vi "CustomEventHandler.vi"(11 "MicronGRPC.lvclass":refnum<class "MicronGRPC.lvclass">) -> ()   [LabVIEW 2019, in "MicronGRPCGeneratedServer.lvlib"]
uses:
  MicronGRPCGeneratedServer.lvlib
  RPC Service/MicronGRPC/MicronGRPC.lvclass
  Message/GRPCMessage.lvclass
  D:/GitHub/KarthikAbiram/Micron/LabVIEW/Source/vi.lib/Micron/Base/Server/Message/MessageBase.lvclass
  <vilib>/SLL Toolkit/SLL String/SLL String.lvlib
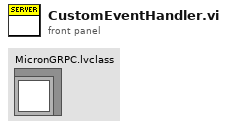
[diagram p1: front panel]
types:
  T1 = typedef "grpc-lvsupport-release.lvlib/grpcId.ctl" = u64
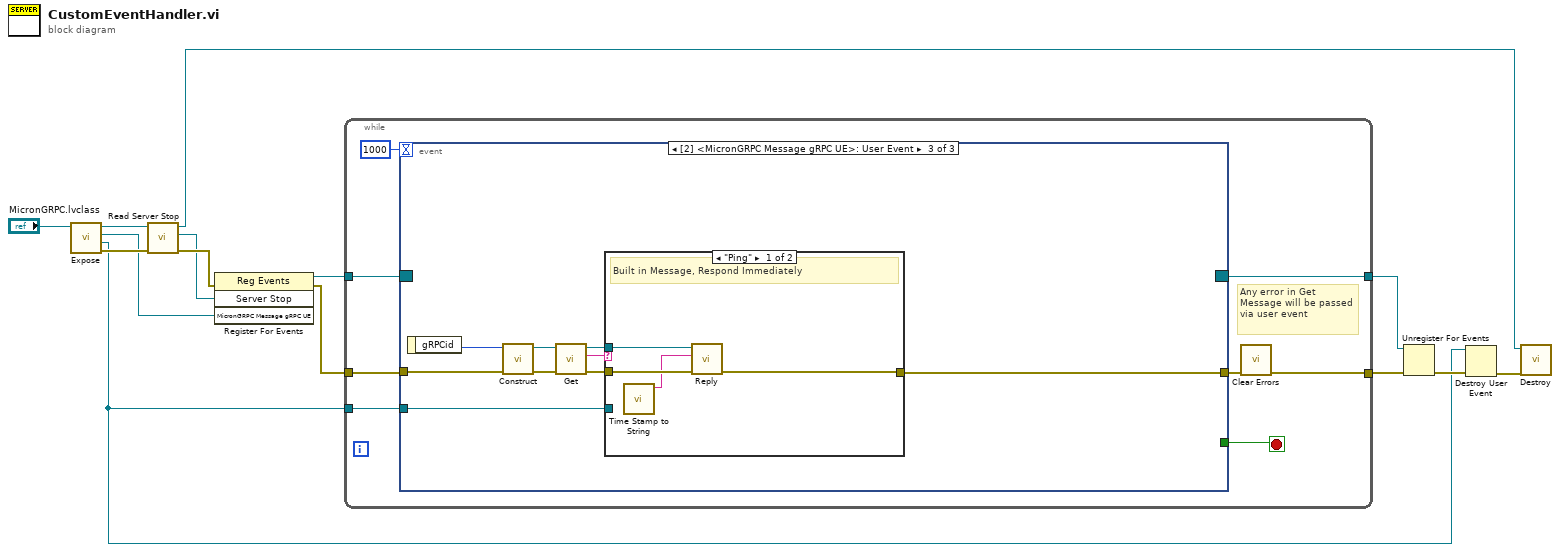
[diagram p0: block diagram]
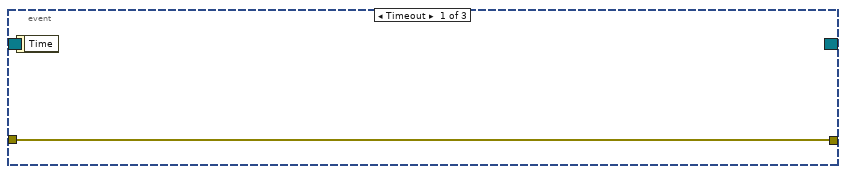
[diagram p2: hidden frame]
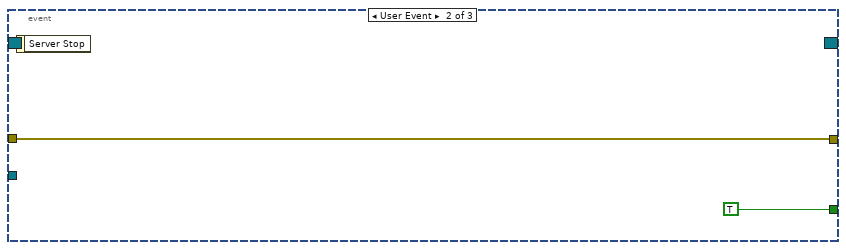
[diagram p3: hidden frame]
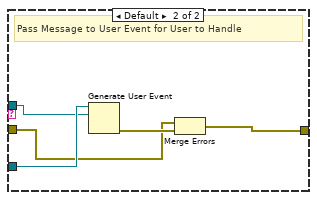
[diagram p4: hidden frame]
diagram:
  n1 = call "Expose.vi"("MicronGRPC in"="MicronGRPC.lvclass") -> ("error out"=w10:errorcluster, "MicronUE"=w4:refnum<user-event>, "MicronGRPC Message gRPC UE"=w9:refnum<user-event>, "MicronGRPC out"=w11:refnum<class "MicronGRPC.lvclass">)  [unwired: 7 in]
  n2 = call-dynamic "Read Server Stop.vi"("error in"=w10, "gRPC service in"=w11) -> ("error out"=w8:errorcluster, "Server Stop"=w3:refnum<user-event>, "gRPC service out"=w2:refnum<class "MicronGRPC.lvclass">)  [unwired: 7 in]
  n3 = register-events(error in=w8, w3, w9) -> (reference out=w14:refnum<event-registration>, error out=w13:errorcluster)  [unwired: 1 in]
  n4 = while {
    tunnel: w14 -> [w22]
    tunnel: [w20] -> w6
    tunnel: w13 -> [w18]
    tunnel: [w15] -> w7
    tunnel: w4 -> [w17]
    stop <- w21 stop-if-true
    # "Any error in Get Message will be passed via user event"
    n5 = event "RPC Methods Event Structure" shown="[2] <MicronGRPC Message gRPC UE>: User Event" {
      selector: w22 -> [_ _ _]
      dyn-events: [_ _ _] -> w20
      timeout: 1000 -> [_ _ _]
      tunnel: [_ TRUE _] -> w21
      tunnel: w18 -> [w23 w24 w33]
      tunnel: [w23 w24 w32] -> w16
      tunnel: w17 -> [_ _ w31]
      event Timeout {
        n6 = event-data() -> ()  [unwired: 1 in, 1 out]
      }
      event User Event {
        n7 = event-data() -> ()  [unwired: 1 in, 1 out]
      }
      event User Event {
        n8 = event-data() -> ("gRPCid"=w34:T1)  [unwired: 1 in]
        n9 = call "Construct.vi"("error in (no error)"=w33, "gRPCid"=w34) -> ("error out"=w29:errorcluster, "GRPCMessage out"=w30:refnum<class "GRPCMessage.lvclass">)  [unwired: 8 in]
        n10 = call-dynamic "Get.vi"("error in (no error)"=w29, "MicronMessage in"=w30) -> ("error out"=w28:errorcluster, "Command"=w27:string, "MicronMessage out"=w26:refnum<class "GRPCMessage.lvclass">)  [unwired: 6 in, 1 out]
        n11 = case shown="\"Ping\"" w27 {
          tunnel: [w36 w40] -> w32
          tunnel: w31 -> [_ w42]
          tunnel: w28 -> [w38 w39]
          tunnel: w26 -> [w37 w41]
          frame "Ping" {
            # "Built in Message, Respond Immediately"
            n12 = call <vilib>:"Time Stamp to String.vi"() -> ("Output String"=w35:string)  [unwired: 11 in]
            n13 = call-dynamic "Reply.vi"("error in (no error)"=w38, "Response"=w35, "MicronMessage in"=w37) -> ("error out"=w36:errorcluster)  [unwired: 7 in, 1 out]
          }
          frame Default {
            # "Pass Message to User Event for User to Handle"
            n14 = Generate User Event(user event=w42, event data cluster=w41) -> (error out=w43:errorcluster)  [unwired: 2 in, 1 out]
            n15 = Merge Errors(w39, w43) -> (w40:errorcluster)
          }
        }
      }
    }
    n16 = call <vilib>:"Clear Errors.vi"("error in (no error)"=w16) -> ("error out"=w15:errorcluster)  [unwired: 5 in, 1 out]
  }
  n17 = Unregister For Events(event registration refnum=w6, error in=w7) -> (error out=w5:errorcluster)
  n18 = Destroy User Event(user event=w4, error in=w5) -> (error out=w1:errorcluster)
  n19 = call-dynamic "Destroy.vi"("error in (no error)"=w1, "SignalGeneratorService in"=w2) -> ()  [unwired: 8 in, 2 out]
